vi "Format Node ID.vi"(11 "node":i32) -> (3 "formatted node ID":string)   [LabVIEW 2015, in "GraphViz Mapping Visualizer.lvlib"]
uses:
  GraphViz Mapping Visualizer.lvlib
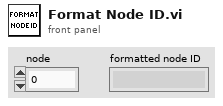
[diagram p1: front panel]
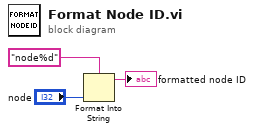
[diagram p0: block diagram]
diagram:
  n1 = Format Into String(format string="node%d", "node") -> (resulting string=→"formatted node ID":string)  [unwired: 2 in, 1 out]
